vi "PC Control.vi"(11 "Queue in":refnum<queue>) -> ()   [LabVIEW 2014]
uses:
  controls/UI DataSam.ctl
  controls/Command Parser Enum.ctl
  controls/Control ConfigurationSam.ctl
  controls/UI Data.ctl
  globals/RT Network Stream Endpoints.vi
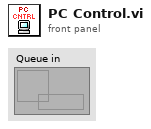
[diagram p1: front panel]
types:
  T1 = typedef "Command Parser Enum.ctl" = enum16{"Initialize", "Listen for Writer", "Receive Commands"}
  T2 = typedef "UI DataSam.ctl" = cluster{"Message":string, "Data":variant}
  T3 = typedef "UI Data.ctl" = cluster{"Message":string, "Data":variant}
  T4 = typedef "Control ConfigurationSam.ctl" = cluster{"PID Gains":cluster{"proportional gain (Kc)":dbl, "integral gain (Kc*Ts/Ti)":dbl, "derivative gain (Kc*Td/Ts)":dbl}, "Output Range":cluster{"output high":dbl, "output low":dbl}}
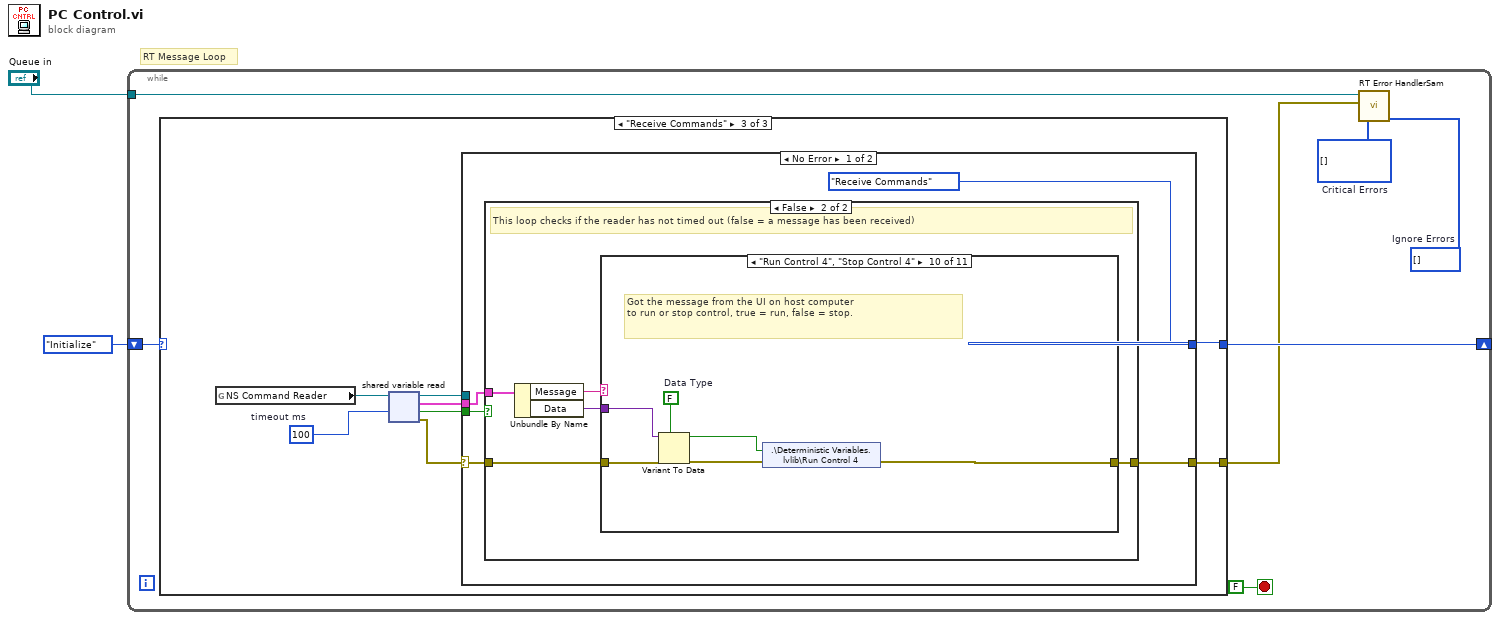
[diagram p0: block diagram]
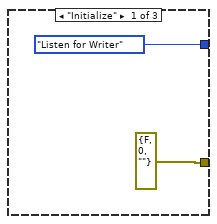
[diagram p2: hidden frame]
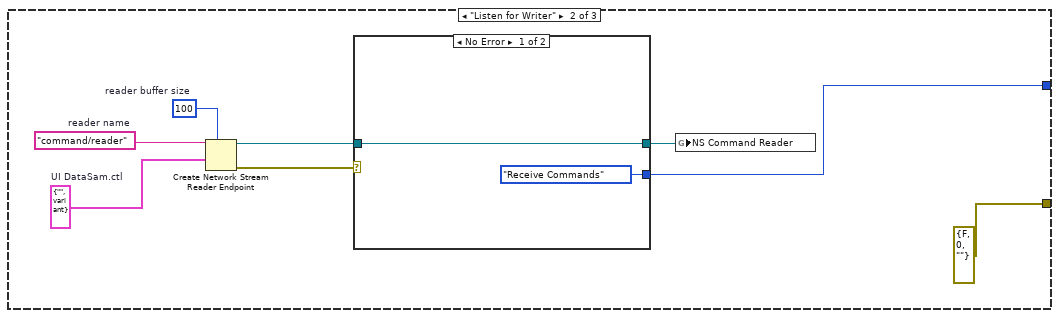
[diagram p3: hidden frame]
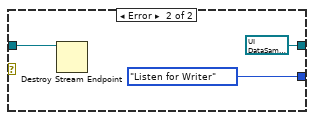
[diagram p4: hidden frame]
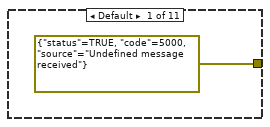
[diagram p6: hidden frame]
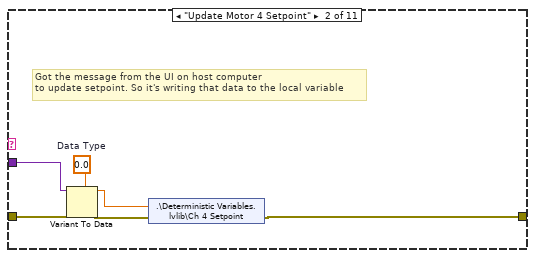
[diagram p7: hidden frame]
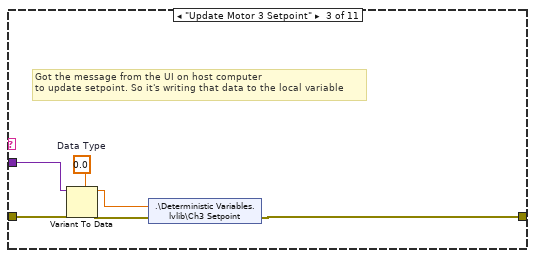
[diagram p8: hidden frame]
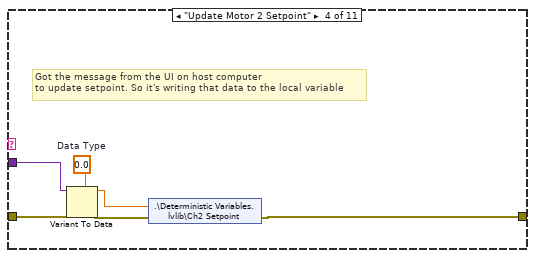
[diagram p9: hidden frame]
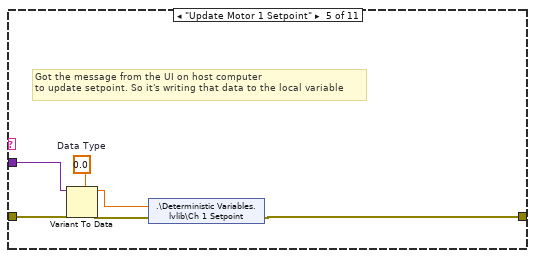
[diagram p10: hidden frame]
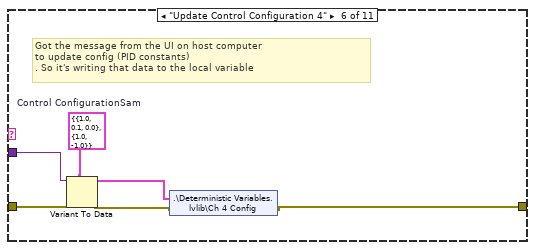
[diagram p11: hidden frame]
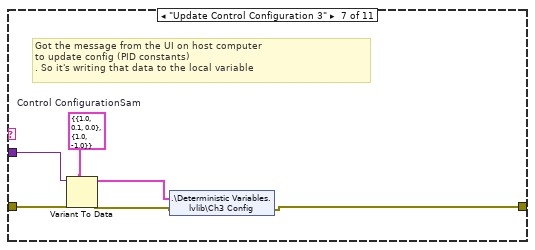
[diagram p12: hidden frame]
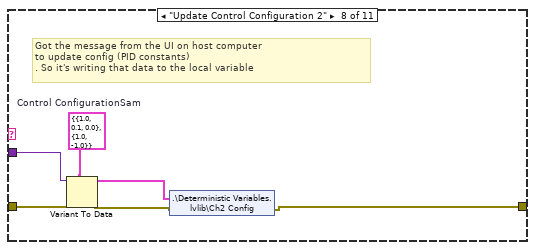
[diagram p13: hidden frame]
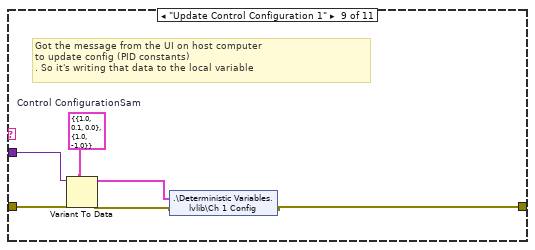
[diagram p14: hidden frame]
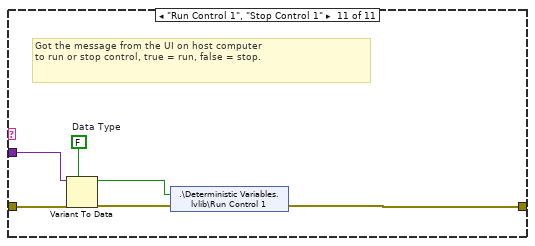
[diagram p15: hidden frame]
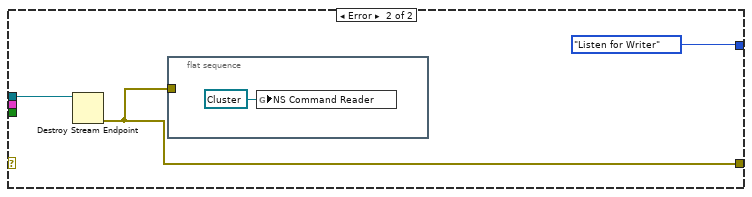
[diagram p16: hidden frame]
diagram:
  # "RT Message Loop"
  n1 = while {
    shift-right: [w7] -> _
    shift-left: Command_Parser_Enum."Initialize" ("Command Parser Enum") -> [w9]
    tunnel: "Queue in" -> [w6]
    stop <- FALSE stop-if-true
    w4 = i32[] []  # Ignore Errors
    w5 = i32[] []  # Critical Errors
    n2 = case shown="\"Receive Commands\"" w9 {
      tunnel: [Command_Parser_Enum."Listen for Writer" ("Command Parser Enum") w15 w26] -> w7
      tunnel: [errorcluster {"status"=FALSE, "code"=0, "source"=""} ("error constant") errorcluster {"status"=FALSE, "code"=0, "source"=""} ("error constant") w25] -> w3
      frame "Initialize" {
      }
      frame "Listen for Writer" {
        w13 = T2 {"Message"="", "Data"=variant}  # UI DataSam.ctl
        w17 = 100  # reader buffer size
        w18 = "command/reader"  # reader name
        n3 = Create Network Stream Reader Endpoint(7:w17, 9:w13, 11:w18) -> (0:w19:errorcluster, 3:w16:refnum<k21>)  [unwired: 4 in]
        n4 = case shown="No Error" w19 {
          tunnel: w16 -> [w20 w22]
          tunnel: [Command_Parser_Enum."Receive Commands" ("Command Parser Enum") Command_Parser_Enum."Listen for Writer" ("Command Parser Enum")] -> w15
          tunnel: [w20 refnum<k21> refnum ("reader name")] -> w12
          frame No Error {
          }
          frame Error {
            n5 = Destroy Stream Endpoint(11:w22) -> ()  [unwired: 1 in, 1 out]
          }
        }
        n6 = global write "RT Network Stream Endpoints.vi" "NS Command Reader"(w12) -> ()
      }
      frame "Receive Commands" {
        w31 = 100  # timeout ms
        n7 = global read "RT Network Stream Endpoints.vi" "NS Command Reader"() -> (w32:refnum<k21>)
        n8 = shared-variable-read(w32, w31) -> (w27:refnum<k21>, w30:errorcluster, w29:bool, w28:T3)  [unwired: 1 in]
        n9 = case shown="No Error" w30 {
          selector: w30 -> [w35 _]
          tunnel: w29 -> [w36 _]
          tunnel: w28 -> [w33 _]
          tunnel: w27 -> [_ w107]
          tunnel: [Command_Parser_Enum."Receive Commands" ("Command Parser Enum") Command_Parser_Enum."Listen for Writer" ("Command Parser Enum")] -> w26
          tunnel: [w34 w106] -> w25
          frame No Error {
            n10 = case shown="False" w36 {
              tunnel: w35 -> [w38 w40]
              tunnel: [w38 w39] -> w34
              tunnel: w33 -> [_ w43]
              frame True {
                # "This loop checks if the reader has not timed out (false = a message has been received)"
              }
              frame False {
                # "This loop checks if the reader has not timed out (false = a message has been received)"
                n11 = Unbundle By Name(w43) -> ("Message"=w42:string, "Data"=w41:variant)
                n12 = case shown="\"Run Control 4\", \"Stop Control 4\"" w42 {
                  tunnel: w41 -> [_ w49 w55 w61 w67 w73 w79 w85 w91 w97 w103]
                  tunnel: w40 -> [_ w50 w56 w62 w68 w74 w80 w86 w92 w98 w104]
                  tunnel: [errorcluster {"status"=TRUE, "code"=5000, "source"="Undefined message received"} ("error IO") w45 w51 w57 w63 w69 w75 w81 w87 w94 w100] -> w39
                  frame Default {
                  }
                  frame "Update Motor 4 Setpoint" {
                    w48 = 0.0  # Data Type
                    # "Got the message from the UI on host computer\nto update setpoint. So it's writing that data to the local variable"
                    n13 = Variant To Data(error in=w50, type=w48, Variant=w49) -> (data=w47:dbl, error out=w46:errorcluster)
                    n14 = shared-variable ".\\Deterministic Variables.lvlib\\Ch 4 Setpoint"(w47, error in=w46) -> (error out=w45:errorcluster)
                  }
                  frame "Update Motor 3 Setpoint" {
                    w54 = 0.0  # Data Type
                    # "Got the message from the UI on host computer\nto update setpoint. So it's writing that data to the local variable"
                    n15 = Variant To Data(error in=w56, type=w54, Variant=w55) -> (data=w53:dbl, error out=w52:errorcluster)
                    n16 = shared-variable ".\\Deterministic Variables.lvlib\\Ch3 Setpoint"(w53, error in=w52) -> (error out=w51:errorcluster)
                  }
                  frame "Update Motor 2 Setpoint" {
                    w60 = 0.0  # Data Type
                    # "Got the message from the UI on host computer\nto update setpoint. So it's writing that data to the local variable"
                    n17 = Variant To Data(error in=w62, type=w60, Variant=w61) -> (data=w59:dbl, error out=w58:errorcluster)
                    n18 = shared-variable ".\\Deterministic Variables.lvlib\\Ch2 Setpoint"(w59, error in=w58) -> (error out=w57:errorcluster)
                  }
                  frame "Update Motor 1 Setpoint" {
                    w66 = 0.0  # Data Type
                    # "Got the message from the UI on host computer\nto update setpoint. So it's writing that data to the local variable"
                    n19 = Variant To Data(error in=w68, type=w66, Variant=w67) -> (data=w65:dbl, error out=w64:errorcluster)
                    n20 = shared-variable ".\\Deterministic Variables.lvlib\\Ch 1 Setpoint"(w65, error in=w64) -> (error out=w63:errorcluster)
                  }
                  frame "Update Control Configuration 4" {
                    w72 = T4 {"PID Gains"={"proportional gain (Kc)"=1.0, "integral gain (Kc*Ts/Ti)"=0.1, "derivative gain (Kc*Td/Ts)"=0.0}, "Output Range"={"output high"=1.0, "output low"=-1.0}}  # Control ConfigurationSam
                    # "Got the message from the UI on host computer\nto update config (PID constants)\n. So it's writing that data to the local variable"
                    n21 = Variant To Data(error in=w74, type=w72, Variant=w73) -> (data=w70:T4, error out=w71:errorcluster)
                    n22 = shared-variable ".\\Deterministic Variables.lvlib\\Ch 4 Config"(w70, error in=w71) -> (error out=w69:errorcluster)
                  }
                  frame "Update Control Configuration 3" {
                    w78 = T4 {"PID Gains"={"proportional gain (Kc)"=1.0, "integral gain (Kc*Ts/Ti)"=0.1, "derivative gain (Kc*Td/Ts)"=0.0}, "Output Range"={"output high"=1.0, "output low"=-1.0}}  # Control ConfigurationSam
                    # "Got the message from the UI on host computer\nto update config (PID constants)\n. So it's writing that data to the local variable"
                    n23 = Variant To Data(error in=w80, type=w78, Variant=w79) -> (data=w76:T4, error out=w77:errorcluster)
                    n24 = shared-variable ".\\Deterministic Variables.lvlib\\Ch3 Config"(w76, error in=w77) -> (error out=w75:errorcluster)
                  }
                  frame "Update Control Configuration 2" {
                    w84 = T4 {"PID Gains"={"proportional gain (Kc)"=1.0, "integral gain (Kc*Ts/Ti)"=0.1, "derivative gain (Kc*Td/Ts)"=0.0}, "Output Range"={"output high"=1.0, "output low"=-1.0}}  # Control ConfigurationSam
                    # "Got the message from the UI on host computer\nto update config (PID constants)\n. So it's writing that data to the local variable"
                    n25 = Variant To Data(error in=w86, type=w84, Variant=w85) -> (data=w82:T4, error out=w83:errorcluster)
                    n26 = shared-variable ".\\Deterministic Variables.lvlib\\Ch2 Config"(w82, error in=w83) -> (error out=w81:errorcluster)
                  }
                  frame "Update Control Configuration 1" {
                    w90 = T4 {"PID Gains"={"proportional gain (Kc)"=1.0, "integral gain (Kc*Ts/Ti)"=0.1, "derivative gain (Kc*Td/Ts)"=0.0}, "Output Range"={"output high"=1.0, "output low"=-1.0}}  # Control ConfigurationSam
                    # "Got the message from the UI on host computer\nto update config (PID constants)\n. So it's writing that data to the local variable"
                    n27 = Variant To Data(error in=w92, type=w90, Variant=w91) -> (data=w88:T4, error out=w89:errorcluster)
                    n28 = shared-variable ".\\Deterministic Variables.lvlib\\Ch 1 Config"(w88, error in=w89) -> (error out=w87:errorcluster)
                  }
                  frame "Run Control 4", "Stop Control 4" {
                    w96 = FALSE  # Data Type
                    # "Got the message from the UI on host computer\nto run or stop control, true = run, false = stop."
                    n29 = Variant To Data(error in=w98, type=w96, Variant=w97) -> (data=w93:bool, error out=w95:errorcluster)
                    n30 = shared-variable ".\\Deterministic Variables.lvlib\\Run Control 4"(w93, error in=w95) -> (error out=w94:errorcluster)
                  }
                  frame "Run Control 1", "Stop Control 1" {
                    w102 = FALSE  # Data Type
                    # "Got the message from the UI on host computer\nto run or stop control, true = run, false = stop."
                    n31 = Variant To Data(error in=w104, type=w102, Variant=w103) -> (data=w99:bool, error out=w101:errorcluster)
                    n32 = shared-variable ".\\Deterministic Variables.lvlib\\Run Control 1"(w99, error in=w101) -> (error out=w100:errorcluster)
                  }
                }
              }
            }
          }
          frame Error {
            n33 = Destroy Stream Endpoint(11:w107) -> (0:w106:errorcluster)  [unwired: 1 in]
            n34 = flat-sequence {
              tunnel: w106 -> [_]
              frame #0 {
                n35 = global write "RT Network Stream Endpoints.vi" "NS Command Reader"(refnum<k21> refnum ("NS Command Reader")) -> ()
              }
            }
          }
        }
      }
    }
    n36 = call "RT Error HandlerSam.vi"("Ignore Errors"=w4, "Critical Errors"=w5, "error to process"=w3, "queue in"=w6) -> ()  [unwired: 7 in, 1 out]
  }
